vi "Untitled 1.vi"() -> ()   [LabVIEW 2014]
panel:
  out "Array":dbl[](array[numeric])
  out "Waveform Chart":dbl[](graph)
  out "test F":dbl
  in  "point":dbl
  in  "Stop":dbl
  in  "Start":dbl
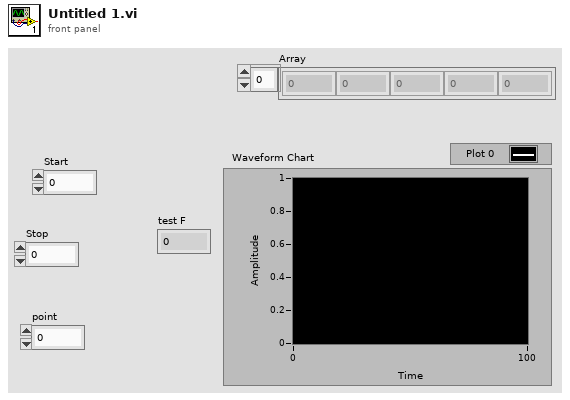
[diagram p1: front panel]
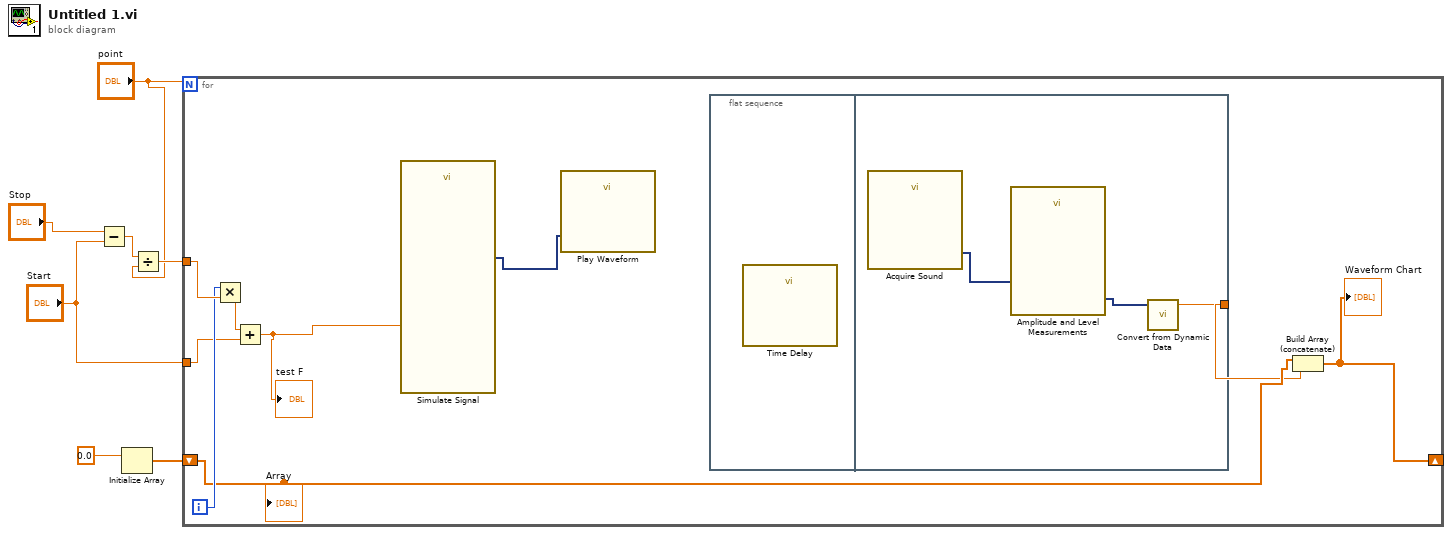
[diagram p0: block diagram]
diagram:
  n1 = Subtract(x="Stop", y="Start") -> (x-y=w6:dbl)
  n2 = Initialize Array(0.0) -> (w2:dbl[])  [unwired: 1 in]
  n3 = Divide(x=w6, y="point") -> (x/y=w4:dbl)
  n4 = for {
    N: "point" -> [_]
    tunnel: "Start" -> [w13]
    tunnel: w4 -> [w15]
    shift-right: [w10] -> _
    shift-left: w2 -> [w12]
    i -> [w14]
    n5 = Multiply(x=w14, y=w15) -> (x*y=w16:dbl)
    n6 = Add(x=w16, y=w13) -> (x+y=w8:dbl)
    "test F" <- w8
    n7 = call "Simulate Signal"("Frequency"=w8) -> ("Sine"=w9:dynamicdata)  [unwired: 13 in, 1 out]
    n8 = call "Play Waveform"("Data"=w9) -> ()  [unwired: 18 in, 1 out]
    n9 = flat-sequence {
      tunnel: [w17] -> w11
      frame #0 {
        n10 = call "Time Delay"() -> ()  [unwired: 11 in, 1 out]
      }
      frame #1 {
        n11 = call "Acquire Sound"() -> ("Data"=w19:dynamicdata)  [unwired: 18 in, 1 out]
        n12 = call "Amplitude and Level Measurements"("Signals"=w19) -> ("Positive Peak"=w18:dynamicdata)  [unwired: 13 in, 1 out]
        n13 = call "Convert from Dynamic Data"("Dynamic Data Type"=w18) -> ("Scalar"=w17:dbl)  [unwired: 3 in]
      }
    }
    n14 = Build Array (concatenate)(w12, w11) -> (w10:dbl[])
    "Waveform Chart" <- w10
    "Array" <- w12
  }
